vi "Result.Report Creator.vi"(2 "Exclude Header CSV":bool, 4 "PassFailResultOnly":bool, 5 "Temp Folder":path, 6 "File Data Objs":T1[](array[typedef]), 7 "Use UUTFolderName":bool, 8 "error in":errorcluster, 9 "Data":T3={"#attributes"={"Version"="MTE_1.0.0"}, "Station"={"Name"="", "PN"="", "SN"="", "Rev"="", "PC Name"="", "Location"="", "HW_Config"={"HW_Item"=[]}, "SW_Config"={"SW_Item"=[]}}, "Test Run"={"Operator"="", "Start Time"=timestamp(0 s since 1904-01-01), "Duration(s)"=0.0, "Mode"="", "Comment"="", "ProcessStep"=""}, "Test Sequence"={"Name"="", "Config"={"Config_Item"=[]}}, "UUTs"={"UUT"=[]}} {"UUTs"."UUT"."Measurements"."Measurement"."Status" items=["LOG", "PASS", "FAIL", "ERROR"]}, 10 "Format":T2, 11 "OutputDir":path) -> (0 "error out":errorcluster, 3 "Output File":path)   [LabVIEW 2018]
uses:
  Result XML/TestResult.FullResultData.ctl
  Result XML/TestResult.Station Info.ctl
  Result XML/TestResult.HW Item.ctl
  Result XML/TestResult.SW Item.ctl
  Result XML/TestResult.Test Run Info.ctl
  Result XML/TestResult.Test Info.ctl
  Result XML/TestResult.UUT Result.ctl
  Result XML/TestResult.Symptom.ctl
  Result XML/TestResult.Symptom.State.ctl
  Result.Measurement Item.ctl
  Result.Measurement and Attribute Item Status.ctl
  Result XML/TestResult.UUTInfo.ctl
  Result.Report Format Selector.ctl
  Reports/Report.Result FileDataObject.ctl
  Result.Factory Logix XLink Adapter, Data Prefixes.ctl
  <vilib>/KATE/Files/File Utils.lvlib
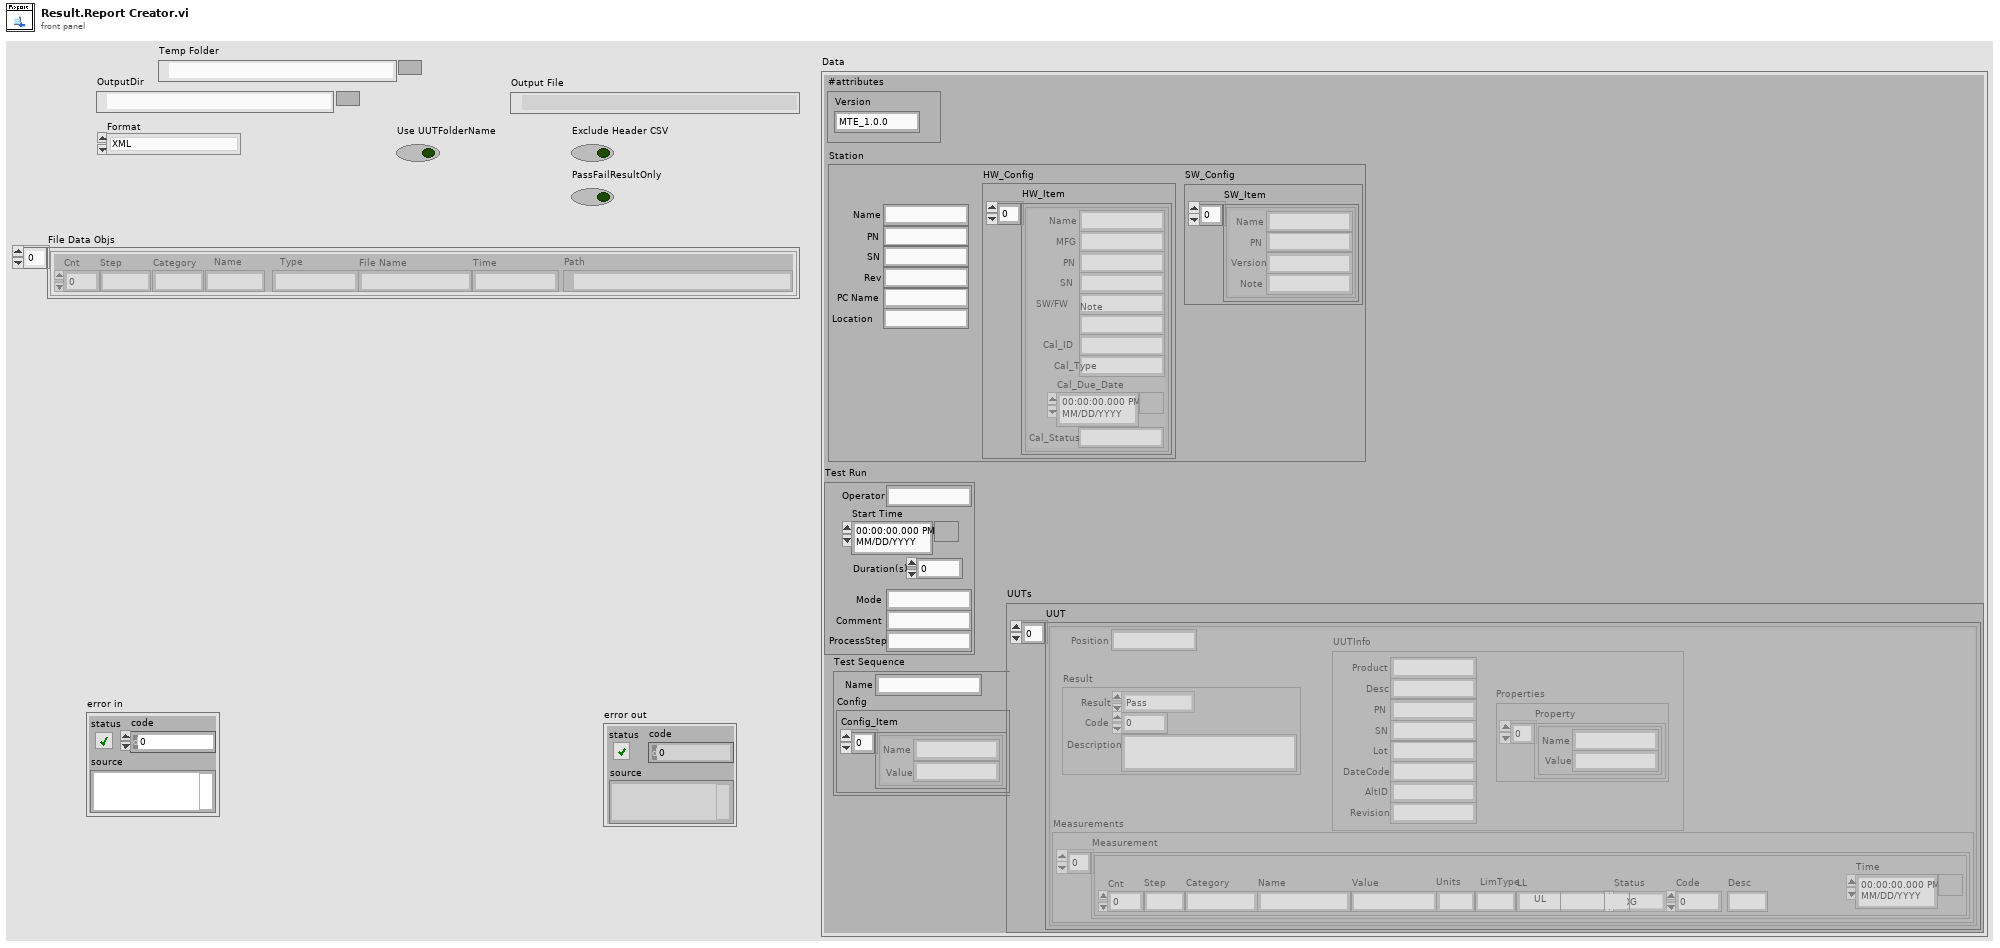
[diagram p1: front panel]
types:
  T1 = typedef "Report.Result FileDataObject.ctl" = cluster{"Cnt":i32, "Step":string, "Category":string, "Name":string, "Type":string, "File Name":string, "Time":string, "Path":path}
  T2 = typedef "Result.Report Format Selector.ctl" = enum16{"XML", "CSV", "Xlink XML", "XML with Files", "JSON", "JSON with Files", "RTF", "SFC1"}
  T3 = typedef "TestResult.FullResultData.ctl" = cluster{"#attributes":cluster{"Version":string}, "Station":T4, "Test Run":T7, "Test Sequence":T8, "UUTs":cluster{"UUT":T9[]}}
  T4 = typedef "TestResult.Station Info.ctl" = cluster{"Name":string, "PN":string, "SN":string, "Rev":string, "PC Name":string, "Location":string, "HW_Config":cluster{"HW_Item":T5[]}, "SW_Config":cluster{"SW_Item":T6[]}}
  T5 = typedef "TestResult.HW Item.ctl" = cluster{"Name":string, "MFG":string, "PN":string, "SN":string, "SW/FW":string, "Note":string, "Cal_ID":string, "Cal_Type":string, "Cal_Due_Date":timestamp, "Cal_Status":string}
  T6 = typedef "TestResult.SW Item.ctl" = cluster{"Name":string, "PN":string, "Version":string, "Note":string}
  T7 = typedef "TestResult.Test Run Info.ctl" = cluster{"Operator":string, "Start Time":timestamp, "Duration(s)":dbl, "Mode":string, "Comment":string, "ProcessStep":string}
  T8 = typedef "TestResult.Test Info.ctl" = cluster{"Name":string, "Config":cluster{"Config_Item":cluster{"Name":string, "Value":string}[]}}
  T9 = typedef "TestResult.UUT Result.ctl" = cluster{"Position":string, "Result":T10, "Measurements":cluster{"Measurement":T12[]}, "UUTInfo":T14}
  T10 = typedef "TestResult.Symptom.ctl" = cluster{"Result":T11, "Code":i32, "Description":string}
  T11 = typedef "TestResult.Symptom.State.ctl" = enum16{"Pass", "Fail", "Error", "Aborted", "Completed", "Logged"}
  T12 = typedef "Result.Measurement Item.ctl" = cluster{"Cnt":i32, "Step":string, "Category":string, "Name":string, "Value":string, "Units":string, "LimType":string, "LL":string, "UL":string, "Status":T13, "Code":i32, "Desc":string, "Time":timestamp}
  T13 = typedef "Result.Measurement and Attribute Item Status.ctl" = i32
  T14 = typedef "TestResult.UUTInfo.ctl" = cluster{"Product":string, "Desc":string, "PN":string, "SN":string, "Lot":string, "DateCode":string, "AltID":string, "Revision":string, "Properties":cluster{"Property":cluster{"Name":string, "Value":string}[]}}
  T15 = typedef "Result.Factory Logix XLink Adapter, Data Prefixes.ctl" = cluster{"Test Run":string, "Client Setup":string, "Client SW":string, "Client HW":string, "Attribute":string, "Numeric":string, "Client ID":string}
  T16 = cluster{"OutputDir":path, "File Data Objs":T1[], "Output File":path, "Format":T2, "File Name":string, "Station":T4, "Test Run":T7, "Test Sequence":T8, "UUT":T9}
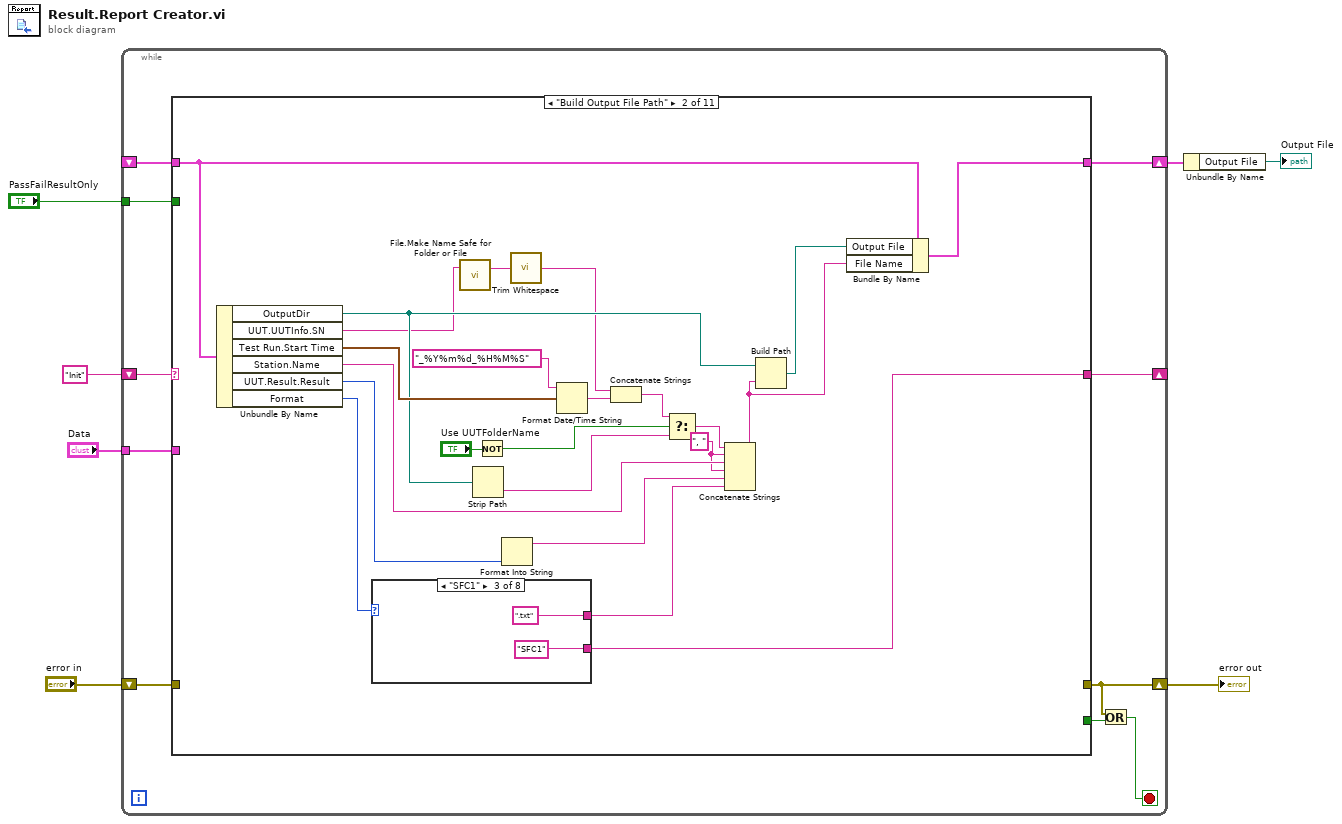
[diagram p0: block diagram]
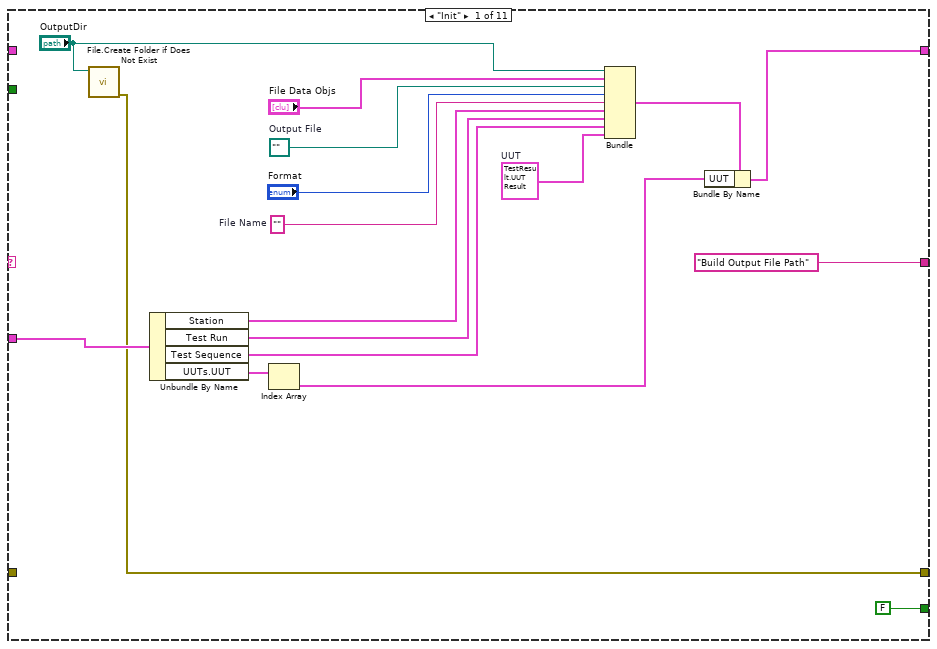
[diagram p2: hidden frame]
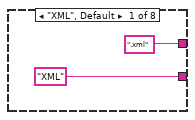
[diagram p3: hidden frame]
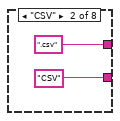
[diagram p4: hidden frame]
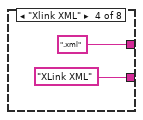
[diagram p5: hidden frame]
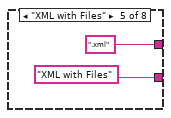
[diagram p6: hidden frame]
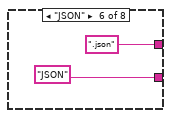
[diagram p7: hidden frame]
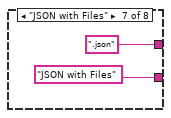
[diagram p8: hidden frame]
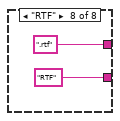
[diagram p9: hidden frame]
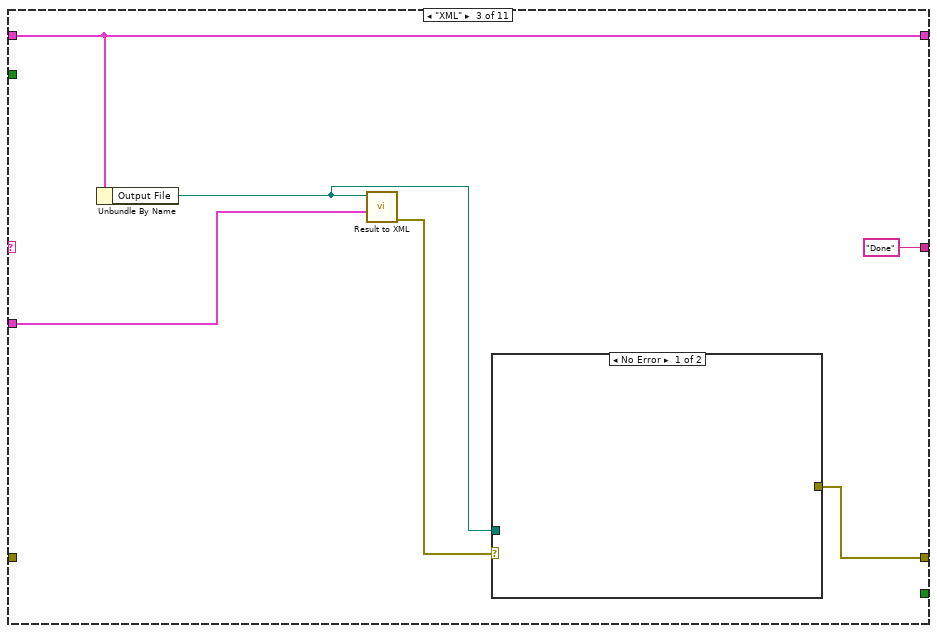
[diagram p10: hidden frame]
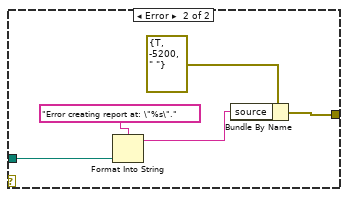
[diagram p11: hidden frame]
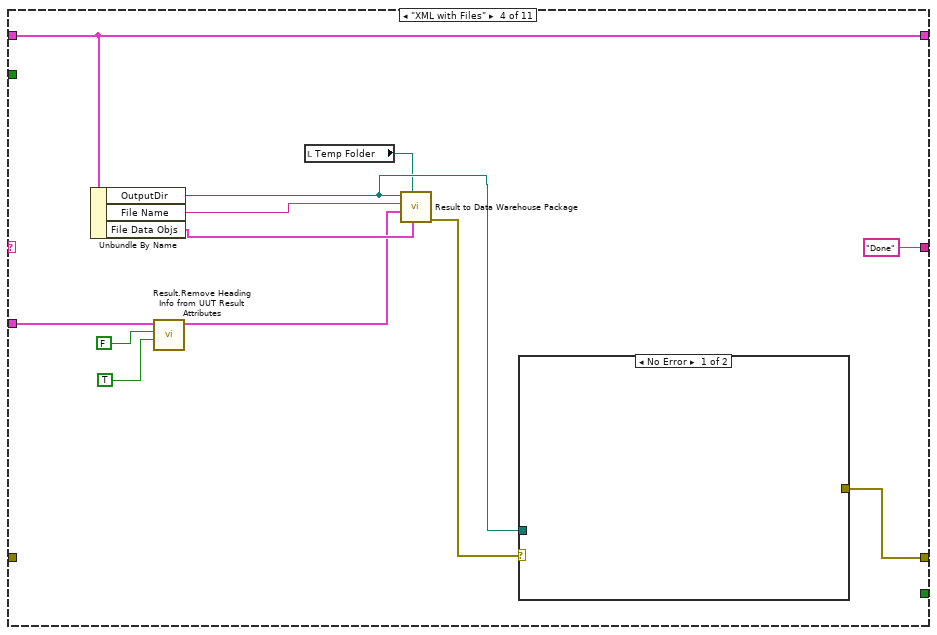
[diagram p12: hidden frame]
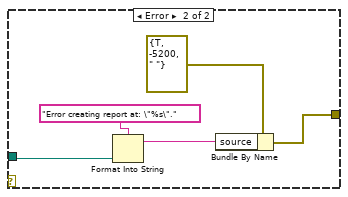
[diagram p13: hidden frame]
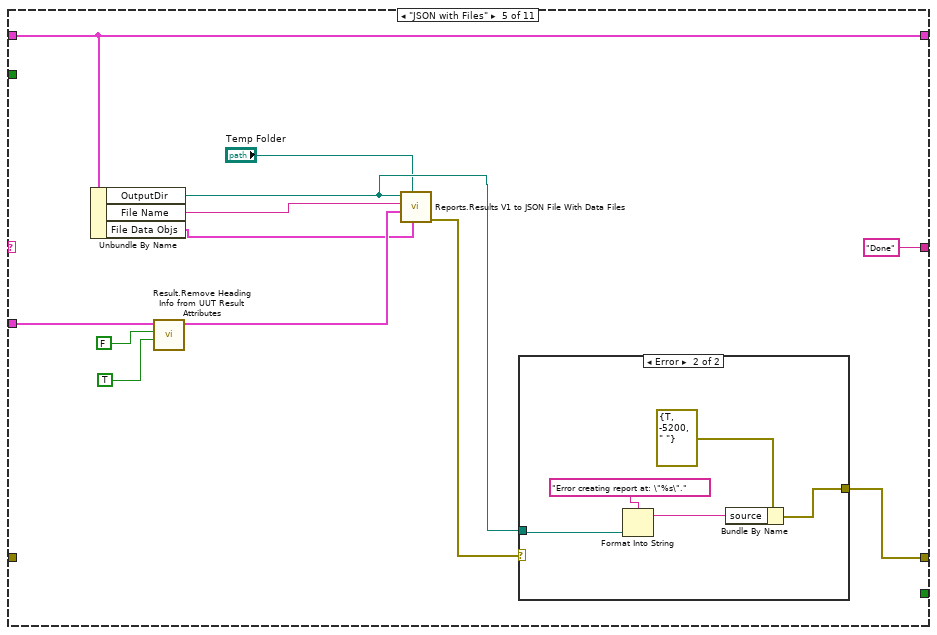
[diagram p14: hidden frame]
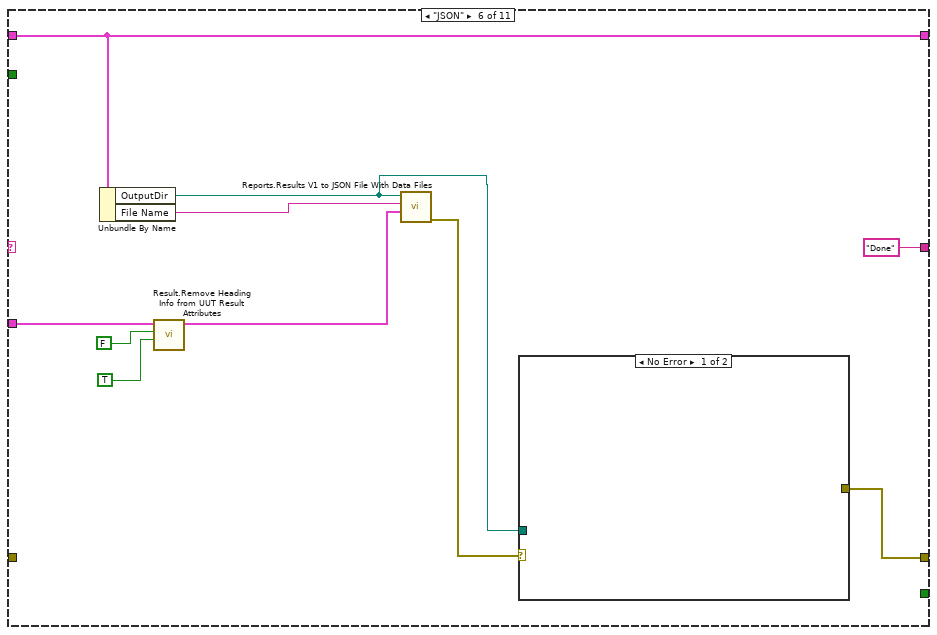
[diagram p16: hidden frame]
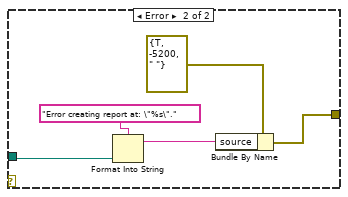
[diagram p17: hidden frame]
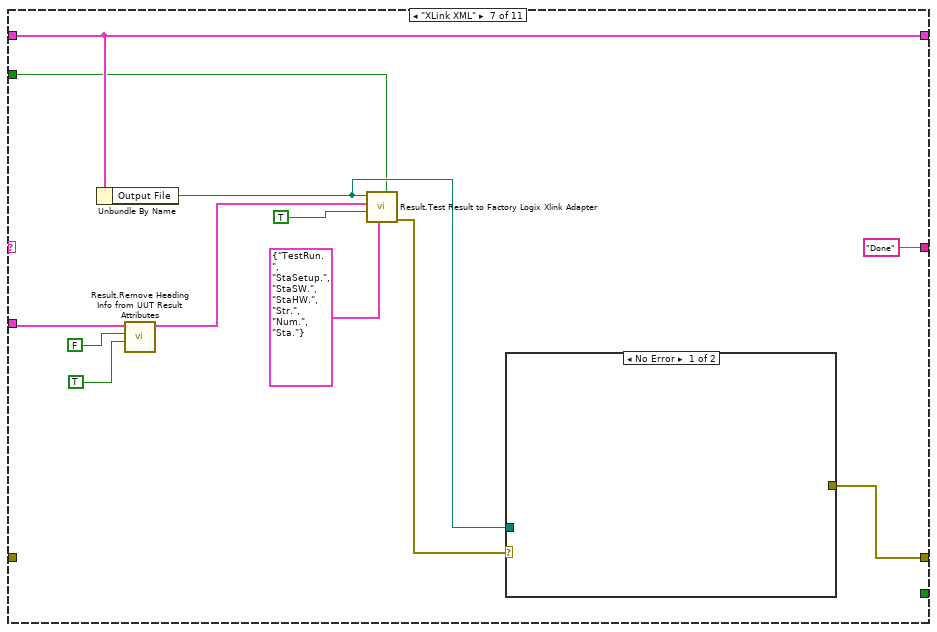
[diagram p18: hidden frame]
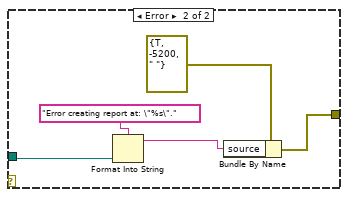
[diagram p19: hidden frame]
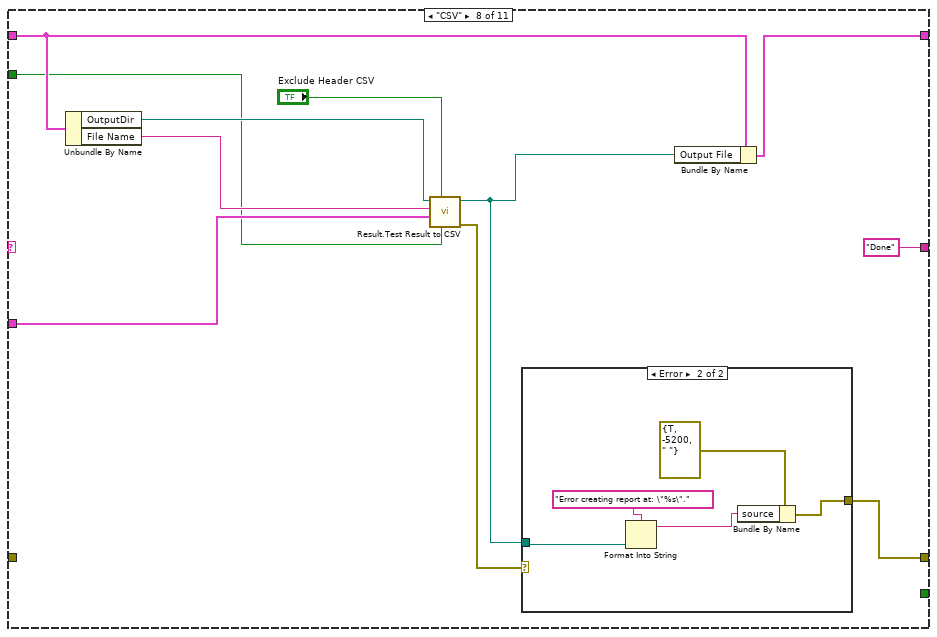
[diagram p20: hidden frame]
diagram:
  n1 = while {
    shift-right: [w11] -> w4
    shift-left: _ -> [w12]
    shift-right: [w10] -> _
    shift-left: "Init" -> [w17]
    shift-right: [w15] -> w5
    shift-left: "error in" -> [w16]
    tunnel: "Data" -> [w9]
    tunnel: "PassFailResultOnly" -> [w8]
    stop <- w13 stop-if-true
    n2 = case shown="\"Build Output File Path\"" w17 {
      tunnel: w16 -> [_ _ _ _ _ _ _ _ _ _ _]
      tunnel: [w19 _ w74 w90 w108 w123 w143 w153 w167 _ _] -> w15
      tunnel: [FALSE _ _ _ _ _ _ _ _ _ TRUE] -> w14
      tunnel: w12 -> [_ w56 w79 w96 w113 w128 w145 w157 w171 w182 w186]
      tunnel: [w22 w57 w79 w96 w113 w128 w145 w156 w170 w182 w185] -> w11
      tunnel: ["Build Output File Path" w50 "Done" "Done" "Done" "Done" "Done" "Done" "Done" "Done" _] -> w10
      tunnel: w9 -> [w20 _ w77 w89 w107 w122 w138 w158 w172 _ _]
      tunnel: w8 -> [_ _ _ _ _ _ w134 w151 _ _ _]
      frame "Init" {
        w21 = ""  # File Name
        w25 = T9 {"Position"="", "Result"={"Result"=enum."Pass", "Code"=0, "Description"=""}, "Measurements"={"Measurement"=[]}, "UUTInfo"={"Product"="", "Desc"="", "PN"="", "SN"="", "Lot"="", "DateCode"="", "AltID"="", "Revision"="", "Properties"={"Property"=[]}}}  # UUT
        w32 = path ""  # Output File
        n3 = call <vilib>:"File.Create Folder if Does Not Exist.vi"("Path"="OutputDir") -> ("error out"=w19:errorcluster)  [unwired: 8 in, 2 out]
        n4 = Unbundle By Name(w20) -> ("Station"=w28:T4, "Test Run"=w27:T7, "Test Sequence"=w26:T8, "UUTs.UUT"=w29:T9[])
        n5 = Index Array(array=w29) -> (element=w24:T9)  [unwired: 1 in]
        n6 = Bundle("OutputDir"="OutputDir", "File Data Objs"="File Data Objs", "Output File"=w32, "Format"="Format", "File Name"=w21, "Station"=w28, "Test Run"=w27, "Test Sequence"=w26, "UUT"=w25) -> (w23:T16)  [unwired: 1 in]
        n7 = Bundle By Name(cluster=w23, "UUT"=w24) -> (w22:T16)
      }
      frame "Build Output File Path" {
        w40 = ", "
        n8 = Unbundle By Name(w56) -> ("OutputDir"=w49:path, "UUT.UUTInfo.SN"=w37:string, "Test Run.Start Time"=w53:timestamp, "Station.Name"=w48:string, "UUT.Result.Result"=w39:T11, "Format"=w52:T2)
        n9 = case shown="\"SFC1\"" w52 {
          tunnel: [".xml" ".csv" ".txt" ".xml" ".xml" ".json" ".json" ".rtf"] -> w41
          tunnel: ["XML" "CSV" "SFC1" "XLink XML" "XML with Files" "JSON" "JSON with Files" "RTF"] -> w50
          frame "XML", Default {
          }
          frame "CSV" {
          }
          frame "SFC1" {
          }
          frame "Xlink XML" {
          }
          frame "XML with Files" {
          }
          frame "JSON" {
          }
          frame "JSON with Files" {
          }
          frame "RTF" {
          }
        }
        n10 = call <vilib>:"File.Make Name Safe for Folder or File.vi"("File Name"=w37) -> ("Fixed Name"=w36:string)  [unwired: 2 in]
        n11 = Strip Path(path=w49) -> (name=w43:string)  [unwired: 1 out]
        n12 = Not(x="Use UUTFolderName") -> (.not. x?=w44:bool)
        n13 = Format Into String(w39) -> (resulting string=w38:string)  [unwired: 3 in, 1 out]
        n14 = call <vilib>:"Trim Whitespace.vi"("string"=w36) -> ("trimmed string"=w35:string)  [unwired: 1 in]
        n15 = Format Date/Time String(time format string (%c)="_%Y%m%d_%H%M%S", seconds (now)=w53) -> (date/time string=w55:string)  [unwired: 1 in]
        n16 = Concatenate Strings(w35, w55) -> (w46:string)
        n17 = Select(t=w46, s=w44, f=w43) -> (s? t:f=w47:string)
        n18 = Concatenate Strings(w47, w40, w48, w40, w38, w41) -> (w42:string)
        n19 = Build Path(base path=w49, name or relative path=w42) -> (appended path=w51:path)
        n20 = Bundle By Name(cluster=w56, "Output File"=w51, "File Name"=w42) -> (w57:T16)
      }
      frame "XML" {
        n21 = Unbundle By Name(w79) -> ("Output File"=w76:path)
        n22 = call "Result to XML.vi"("Test Result"=w77, "Path"=w76) -> ("error out"=w75:errorcluster)  [unwired: 9 in]
        n23 = case shown="No Error" w75 {
          tunnel: w76 -> [_ w82]
          tunnel: [_ w81] -> w74
          frame No Error {
          }
          frame Error {
            n24 = Format Into String(format string="Error creating report at: \"%s\"." ("source"), w82) -> (resulting string=w80:string)  [unwired: 2 in, 1 out]
            n25 = Bundle By Name(cluster=errorcluster {"status"=TRUE, "code"=-5200, "source"=" "} ("error constant"), "source"=w80) -> (w81:errorcluster)
          }
        }
      }
      frame "XML with Files" {
        n26 = Unbundle By Name(w96) -> ("OutputDir"=w91:path, "File Name"=w93:string, "File Data Objs"=w94:T1[])
        n27 = call "Result.Remove Heading Info from UUT Result Attributes.vi"("Remove Heading Values"=TRUE, "Remove Headings"=FALSE, "Data"=w89) -> ("Data Out"=w88:T3)  [unwired: 8 in]
        n28 = local read "Temp Folder"() -> (w85:path)
        n29 = call "Result to Data Warehouse Package.vi"("File Data Objs"=w94, "Temp Folder"=w85, "Test Result"=w88, "File Name"=w93, "Folder"=w91) -> ("error out"=w92:errorcluster)  [unwired: 6 in]
        n30 = case shown="No Error" w92 {
          tunnel: [_ w99] -> w90
          tunnel: w91 -> [_ w98]
          frame No Error {
          }
          frame Error {
            n31 = Format Into String(format string="Error creating report at: \"%s\"." ("source"), w98) -> (resulting string=w97:string)  [unwired: 2 in, 1 out]
            n32 = Bundle By Name(cluster=errorcluster {"status"=TRUE, "code"=-5200, "source"=" "} ("error constant"), "source"=w97) -> (w99:errorcluster)
          }
        }
      }
      frame "JSON with Files" {
        n33 = Unbundle By Name(w113) -> ("OutputDir"=w109:path, "File Name"=w111:string, "File Data Objs"=w102:T1[])
        n34 = call "Result.Remove Heading Info from UUT Result Attributes.vi"("Remove Heading Values"=TRUE, "Remove Headings"=FALSE, "Data"=w107) -> ("Data Out"=w103:T3)  [unwired: 8 in]
        n35 = call "Reports.Results V1 to JSON File With Data Files.vi"("File Data Objs"=w102, "Temp Folder"="Temp Folder", "Test Result In"=w103, "File Name"=w111, "Folder"=w109) -> ("error out"=w110:errorcluster)  [unwired: 6 in]
        n36 = case shown="Error" w110 {
          tunnel: [_ w116] -> w108
          tunnel: w109 -> [_ w115]
          frame No Error {
          }
          frame Error {
            n37 = Format Into String(format string="Error creating report at: \"%s\"." ("source"), w115) -> (resulting string=w114:string)  [unwired: 2 in, 1 out]
            n38 = Bundle By Name(cluster=errorcluster {"status"=TRUE, "code"=-5200, "source"=" "} ("error constant"), "source"=w114) -> (w116:errorcluster)
          }
        }
      }
      frame "JSON" {
        n39 = Unbundle By Name(w128) -> ("OutputDir"=w124:path, "File Name"=w126:string)
        n40 = call "Result.Remove Heading Info from UUT Result Attributes.vi"("Remove Heading Values"=TRUE, "Remove Headings"=FALSE, "Data"=w122) -> ("Data Out"=w119:T3)  [unwired: 8 in]
        n41 = call "Reports.Results V1 to JSON File With Data Files.vi"("Test Result In"=w119, "File Name"=w126, "Folder"=w124) -> ("error out"=w125:errorcluster)  [unwired: 8 in]
        n42 = case shown="No Error" w125 {
          tunnel: [_ w131] -> w123
          tunnel: w124 -> [_ w130]
          frame No Error {
          }
          frame Error {
            n43 = Format Into String(format string="Error creating report at: \"%s\"." ("source"), w130) -> (resulting string=w129:string)  [unwired: 2 in, 1 out]
            n44 = Bundle By Name(cluster=errorcluster {"status"=TRUE, "code"=-5200, "source"=" "} ("error constant"), "source"=w129) -> (w131:errorcluster)
          }
        }
      }
      frame "XLink XML" {
        n45 = Unbundle By Name(w145) -> ("Output File"=w142:path)
        n46 = call "Result.Remove Heading Info from UUT Result Attributes.vi"("Remove Heading Values"=TRUE, "Remove Headings"=FALSE, "Data"=w138) -> ("Data Out"=w137:T3)  [unwired: 8 in]
        n47 = call "Result.Test Result to Factory Logix Xlink Adapter.vi"("Overall Result Only"=w134, "Prefixes"=T15 {"Test Run"="TestRun.", "Client Setup"="StaSetup.", "Client SW"="StaSW.", "Client HW"="StaHW.", "Attribute"="Str.", "Numeric"="Num.", "Client ID"="Sta."}, "Add Prefixes"=TRUE, "Test Result"=w137, "Path"=w142) -> ("error out"=w141:errorcluster)  [unwired: 6 in]
        n48 = case shown="No Error" w141 {
          tunnel: [_ w148] -> w143
          tunnel: w142 -> [_ w147]
          frame No Error {
          }
          frame Error {
            n49 = Format Into String(format string="Error creating report at: \"%s\"." ("source"), w147) -> (resulting string=w146:string)  [unwired: 2 in, 1 out]
            n50 = Bundle By Name(cluster=errorcluster {"status"=TRUE, "code"=-5200, "source"=" "} ("error constant"), "source"=w146) -> (w148:errorcluster)
          }
        }
      }
      frame "CSV" {
        n51 = Unbundle By Name(w157) -> ("OutputDir"=w160:path, "File Name"=w159:string)
        n52 = call "Result.Test Result to CSV.vi"("SummaryOnly"=w151, "Exclude Header CSV"="Exclude Header CSV", "Test Result"=w158, "File Name"=w159, "Dir"=w160) -> ("error out"=w154:errorcluster, "File Out"=w155:path)  [unwired: 5 in]
        n53 = case shown="Error" w154 {
          tunnel: [_ w164] -> w153
          tunnel: w155 -> [_ w163]
          frame No Error {
          }
          frame Error {
            n54 = Format Into String(format string="Error creating report at: \"%s\"." ("source"), w163) -> (resulting string=w162:string)  [unwired: 2 in, 1 out]
            n55 = Bundle By Name(cluster=errorcluster {"status"=TRUE, "code"=-5200, "source"=" "} ("error constant"), "source"=w162) -> (w164:errorcluster)
          }
        }
        n56 = Bundle By Name(cluster=w157, "Output File"=w155) -> (w156:T16)
      }
      frame "SFC1" {
        n57 = Unbundle By Name(w171) -> ("OutputDir"=w174:path, "File Name"=w173:string)
        n58 = call "Result.Test Result to SFC1.vi"("Test Result"=w172, "File Name"=w173, "Dir"=w174) -> ("error out"=w168:errorcluster, "Report Path"=w169:path)  [unwired: 7 in]
        n59 = case shown="No Error" w168 {
          tunnel: [_ w178] -> w167
          tunnel: w169 -> [_ w177]
          frame No Error {
          }
          frame Error {
            n60 = Format Into String(format string="Error creating report at: \"%s\"." ("source"), w177) -> (resulting string=w176:string)  [unwired: 2 in, 1 out]
            n61 = Bundle By Name(cluster=errorcluster {"status"=TRUE, "code"=-5200, "source"=" "} ("error constant"), "source"=w176) -> (w178:errorcluster)
          }
        }
        n62 = Bundle By Name(cluster=w171, "Output File"=w169) -> (w170:T16)
      }
      frame "RTF" {
        # "TODO - Add"
        n63 = Unbundle By Name(w182) -> ()  [unwired: 1 out]
      }
      frame "Done", Default {
        # "Empty data - less memory used."
        n64 = Bundle By Name(cluster=w186, "UUT"=T9 {"Position"="", "Result"={"Result"=enum."Pass", "Code"=0, "Description"=""}, "Measurements"={"Measurement"=[]}, "UUTInfo"={"Product"="", "Desc"="", "PN"="", "SN"="", "Lot"="", "DateCode"="", "AltID"="", "Revision"="", "Properties"={"Property"=[]}}}) -> (w185:T16)
      }
    }
    n65 = Or(x=w15, y=w14) -> (x .or. y?=w13:bool)
  }
  "error out" <- w5
  n66 = Unbundle By Name(w4) -> ("Output File"=→"Output File":path)
